vi "Coord window-Build menu.vi"(8 "error in (no error)":errorcluster, 11 "menu":refnum<k9>) -> (0 "error out":errorcluster, 3 "menu reference out":refnum<k9>)   [LabVIEW 2020]
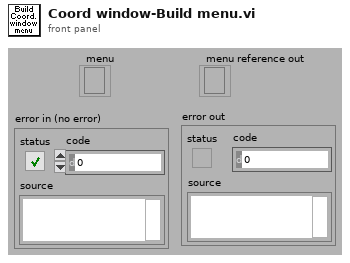
[diagram p1: front panel]
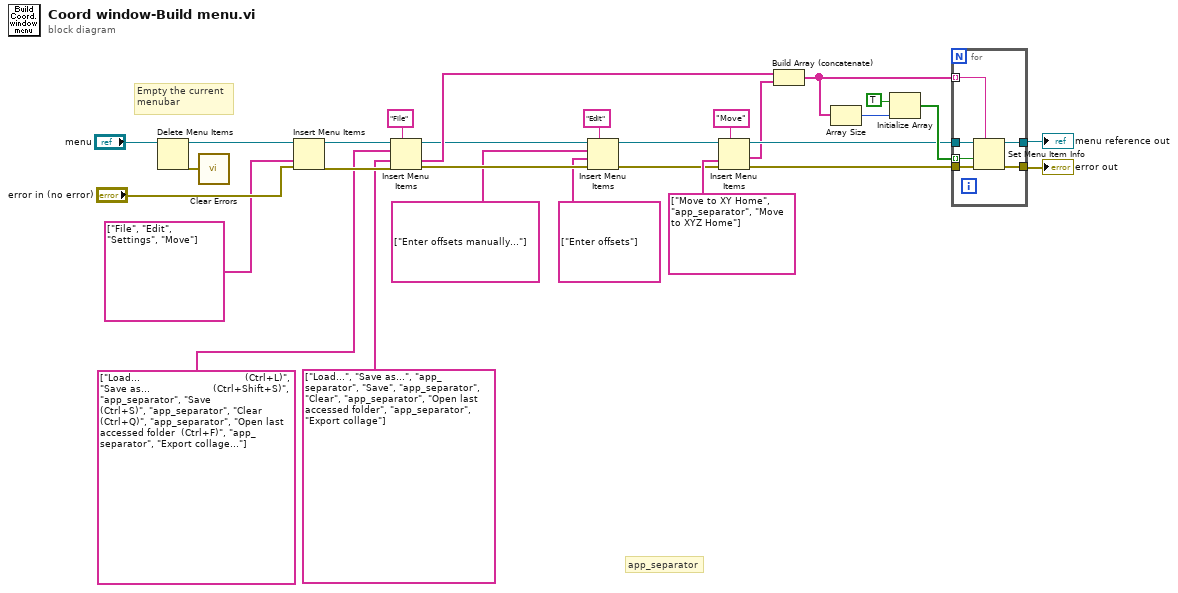
[diagram p0: block diagram]
diagram:
  # "app_separator"
  # "Empty the current\nmenubar"
  n1 = Delete Menu Items(9:"menu") -> (0:w23:errorcluster, 3:w26:refnum<k9>)  [unwired: 2 in, 1 out]
  n2 = call <vilib>:"Clear Errors.vi"("error in (no error)"=w23) -> ()  [unwired: 5 in, 2 out]
  n3 = Insert Menu Items(6:"error in (no error)", 7:string[] ["File", "Edit", "Settings", "Move"] ("item tags"), 9:w26) -> (0:w28:errorcluster, 3:w24:refnum<k9>)  [unwired: 4 out]
  n4 = Insert Menu Items(5:"File" ("menu tag"), 6:w28, 7:string[] ["Load...", "Save as...", "app_separator", "Save", "app_separator", "Clear", "app_separator", "Open last accessed folder", "app_separator", "Export collage"] ("item tags"), 8:string[] ["Load...                                   (Ctrl+L)", "Save as...                     (Ctrl+Shift+S)", "app_separator", "Save                                      (Ctrl+S)", "app_separator", "Clear                                     (Ctrl+Q)", "app_separator", "Open last accessed folder  (Ctrl+F)", "app_separator", "Export collage..."] ("item tags"), 9:w24) -> (0:w5:errorcluster, 1:w20:string[], 3:w6:refnum<k9>)  [unwired: 1 out]
  n5 = Insert Menu Items(5:"Edit" ("menu tag"), 6:w5, 7:string[] ["Enter offsets"] ("item tags"), 8:string[] ["Enter offsets manually..."] ("item tags"), 9:w6) -> (0:w3:errorcluster, 3:w4:refnum<k9>)  [unwired: 2 out]
  n6 = Insert Menu Items(5:"Move" ("menu tag"), 6:w3, 7:string[] ["Move to XY Home", "app_separator", "Move to XYZ Home"] ("item tags"), 9:w4) -> (0:w10:errorcluster, 1:w9:string[], 3:w11:refnum<k9>)  [unwired: 2 out]
  n7 = Build Array (concatenate)(w20, w9) -> (w15:string[])
  n8 = Array Size(array=w15) -> (size(s)=w17:i32)
  n9 = Initialize Array(TRUE, w17) -> (w16:bool[])
  n10 = for {
    tunnel: w11 -> [w35]
    tunnel: [w34] -> w25
    tunnel: w15 -> [w33] mode=indexing
    tunnel: w10 -> [w32]
    tunnel: [w31] -> w29
    tunnel: w16 -> [w30] mode=indexing
    n11 = Set Menu Item Info(7:w33, 8:w32, 9:w30, 11:w35) -> (0:w31:errorcluster, 3:w34:refnum<k9>)  [unwired: 1 in, 2 out]
  }
  "error out" <- w29
  "menu reference out" <- w25
